vi "AppendWaveformRead.vi"(10 "WFM in":T1, 11 "index of element":i32) -> (2 "WFM out":T1, 3 "x = y?":bool)   [LabVIEW 2016, in "system.lvclass"]
uses:
  system.lvclass
  DAQ/Typedefs/PublicEvents--DAQ.Read.ctl
  DAQ/DAQ.lvclass
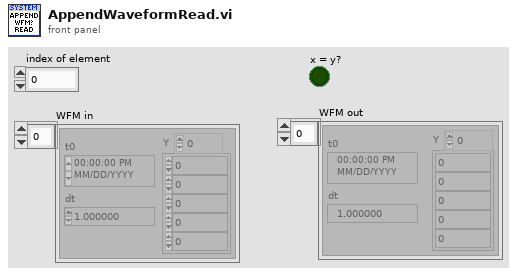
[diagram p1: front panel]
types:
  T1 = typedef "DAQ.lvclass/PublicEvents--DAQ.Read.ctl" = waveform(dbl)[]
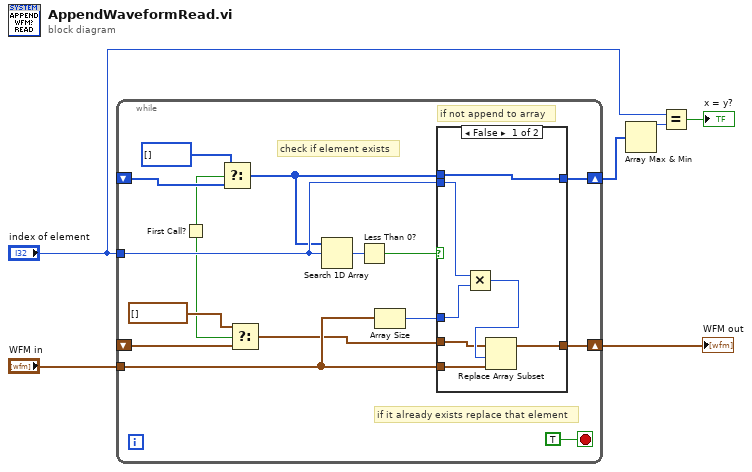
[diagram p0: block diagram]
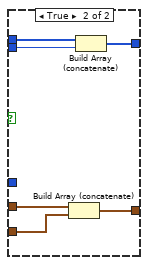
[diagram p2: hidden frame]
diagram:
  n1 = while {
    tunnel: "WFM in" -> [w15]
    tunnel: "index of element" -> [w19]
    shift-right: [w20] -> w4
    shift-left: _ -> [w9]
    shift-right: [w17] -> w5
    shift-left: _ -> [w12]
    stop <- TRUE stop-if-true
    # "if not append to array"
    # "check if element exists"
    # "if it already exists replace that element"
    n2 = First Call?() -> (First Call?: T/F=w7:bool)
    n3 = Select(t=i32[] [], s=w7, f=w9) -> (s? t:f=w8:i32[])
    n4 = Select(t=T1 [], s=w7, f=w12) -> (s? t:f=w11:T1)
    n5 = Search 1D Array(1D array=w8, element=w19) -> (index of element=w18:i32)  [unwired: 1 in]
    n6 = Less Than 0?(x=w18) -> (x < 0?=w16:bool)
    n7 = Array Size(array=w15) -> (size(s)=w14:i32)
    n8 = case shown="False" w16 {
      tunnel: [w23 w34] -> w20
      tunnel: w19 -> [w26 w33]
      tunnel: w8 -> [w23 w32]
      tunnel: w15 -> [w28 w31]
      tunnel: [w27 w30] -> w17
      tunnel: w11 -> [w22 w29]
      tunnel: w14 -> [w25 _]
      frame False {
        n9 = Multiply(x=w26, y=w25) -> (x*y=w24:i32)
        n10 = Replace Array Subset(array=w22, new element=w28, index=w24) -> (w27:T1)
      }
      frame True {
        n11 = Build Array (concatenate)(w29, w31) -> (w30:T1)
        n12 = Build Array (concatenate)(w32, w33) -> (w34:i32[])
      }
    }
  }
  "WFM out" <- w5
  n13 = Array Max & Min(array=w4) -> (max value=w3:i32)  [unwired: 3 out]
  n14 = Equal?(x="index of element", y=w3) -> (x = y?=→"x = y?":bool)
